vi "GetInputs.vi"(8 "Error In":errorcluster, 11 "Pattern Node In":refnum<k20>) -> (0 "Error Out":errorcluster, 2 "Inputs":cluster{"ID":string, "Label":string}[](array[cluster]), 3 "Pattern Node Out":refnum<k20>)   [LabVIEW 2012, in "Virtual-PGA.lvlib"]
uses:
  Virtual-PGA.lvlib
  <vilib>/xml/NI_XML.lvlib
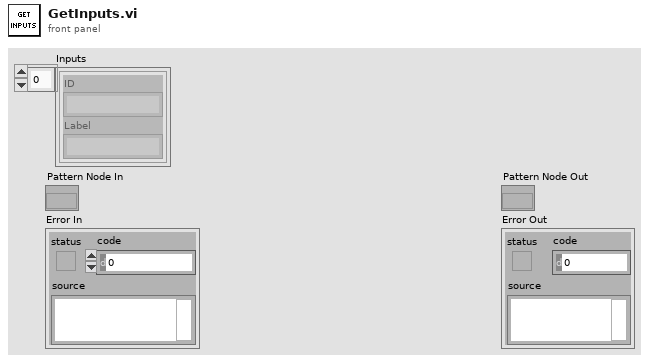
[diagram p1: front panel]
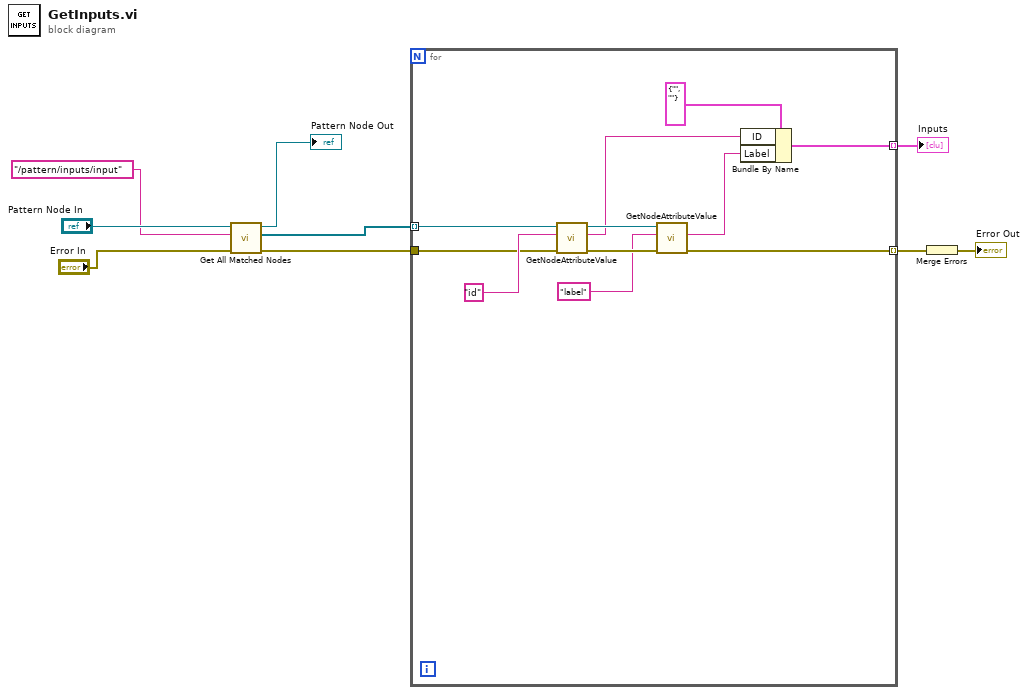
[diagram p0: block diagram]
diagram:
  n1 = call <vilib>:"Get All Matched Nodes.vi"("error in (no error)"="Error In", "XPath expression"="/pattern/inputs/input", "node in"="Pattern Node In") -> ("error out"=w3:errorcluster, "node result array"=w2:refnum<k20>[], "node out"=→"Pattern Node Out":refnum<k20>)  [unwired: 6 in]
  n2 = for {
    tunnel: [w20] -> w9 mode=indexing
    tunnel: w3 -> [w11]
    tunnel: w2 -> [w12] mode=indexing
    tunnel: [w10] -> w1 mode=indexing
    n3 = call "GetNodeAttributeValue.vi"("Error In"=w11, "Attribute Name"="id", "Node In"=w12) -> ("Error Out"=w17:errorcluster, "Value"=w14:string, "Node Out"=w18:refnum<k20>)  [unwired: 6 in]
    n4 = call "GetNodeAttributeValue.vi"("Error In"=w17, "Attribute Name"="label", "Node In"=w18) -> ("Error Out"=w20:errorcluster, "Value"=w13:string)  [unwired: 6 in, 1 out]
    n5 = Bundle By Name(cluster=cluster{"ID":string, "Label":string} {"ID"="", "Label"=""} ("Input"), "ID"=w14, "Label"=w13) -> (w10:cluster{"ID":string, "Label":string})
  }
  "Inputs" <- w1
  n6 = Merge Errors(w9) -> (→"Error Out":errorcluster)
